vi "while_v0_v20.vi"() -> ()   [LabVIEW 2009]
panel:
  out "Waveform Chart":dbl(graph)
  in  "Delay":dbl(slide)=51.42857142857142 scale=0.0..300.0
  out "Out":i64
  in  "stop":bool
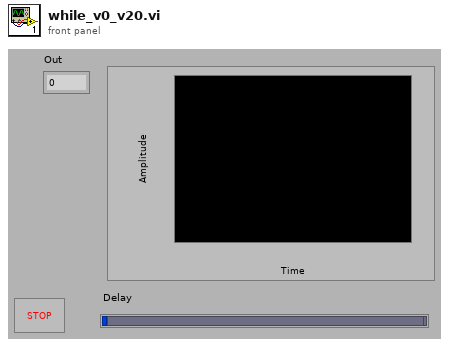
[diagram p1: front panel]
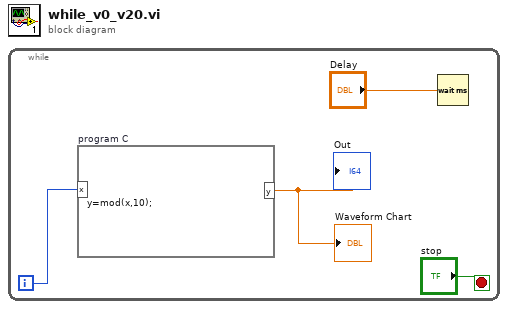
[diagram p0: block diagram]
diagram:
  n1 = while {
    i -> [w2]
    stop <- "stop" stop-if-true
    n2 = formula code="y=mod(x,10);" "program C"("x"=w2) -> ("y"=→"Out" →"Waveform Chart":dbl)
    n3 = Wait (ms)(milliseconds to wait="Delay") -> ()  [unwired: 1 out]
  }
